vi "Buttons.vi"() -> ()   [LabVIEW 2019]
panel:
  in  "Op Buttons":T1={"Align Turret"=9, "Turret Right"=3, "TODO 1"=0, "Turret Left"=1, "Jump Intake"=4, "Shoot"=5, "TODO 2"=11, "TODO 3"=11, "TODO 4"=11, "TODO 5"=11}
  in  "Drive Buttons":T2={"Shift Gear"=9, "Turret Track"=3, "Shoot"=0, "Intake"=1, "Turret Left"=4, "Turret Right"=5, "TODO 2"=11, "TODO 3"=11, "TODO 4"=11, "TODO 5"=11}
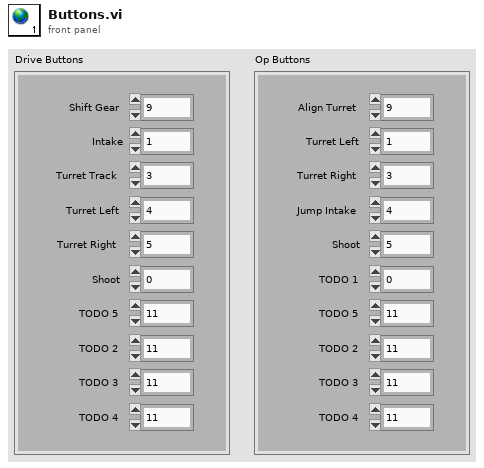
[diagram p1: front panel]
types:
  T1 = cluster{"Align Turret":i32, "Turret Right":i32, "TODO 1":i32, "Turret Left":i32, "Jump Intake":i32, "Shoot":i32, "TODO 2":i32, "TODO 3":i32, "TODO 4":i32, "TODO 5":i32}
  T2 = cluster{"Shift Gear":i32, "Turret Track":i32, "Shoot":i32, "Intake":i32, "Turret Left":i32, "Turret Right":i32, "TODO 2":i32, "TODO 3":i32, "TODO 4":i32, "TODO 5":i32}
diagram:
